vi "Initialize.vi"(8 "error in (no error)":errorcluster, 10 "Variable Names":string[](array[string]), 11 "Expression":string) -> (0 "error out":errorcluster, 3 "Expression":T1)   [LabVIEW 2022 SP3, in "Expressions.lvlib"]
uses:
  Expressions.lvlib
  Controls/Expression.ctl
  Controls/Token Type.ctl
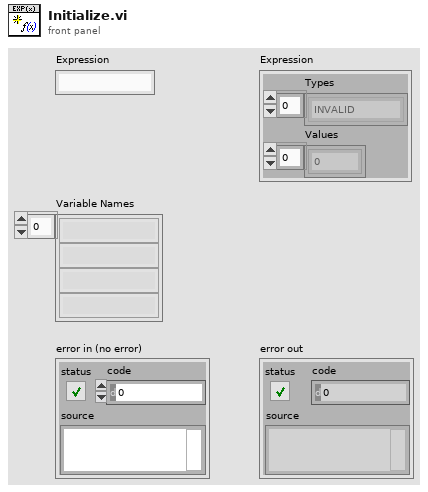
[diagram p1: front panel]
types:
  T1 = typedef "Expressions.lvlib/Expression.ctl" = cluster{"Types":T2[], "Values":dbl[]}
  T2 = typedef "Expressions.lvlib/Token Type.ctl" = enum8{"INVALID", "NOT", "AND", "OR", "EE", "NE", "LT", "GT", "LTE", "GTE", "PLUS", "MINUS", "MULTIPLY", "DIVIDE", "MODULUS", "LPAREN", "RPAREN", "LITERAL", "IDENTIFIER", "DEFINITION"}
  T3 = typedef "Expressions.lvlib/Token.ctl" = cluster{"Offset":i32, "Type":T2, "Value":string}
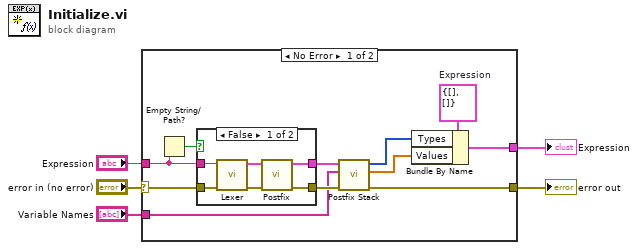
[diagram p0: block diagram]
diagram:
  n1 = case shown="No Error" "error in (no error)" {
    selector: "error in (no error)" -> [w16 w24]
    tunnel: "Expression" -> [w15 _]
    tunnel: "Variable Names" -> [w8 _]
    tunnel: [w10 w24] -> w2
    tunnel: [w12 _] -> w1
    frame No Error {
      w14 = T1 {"Types"=[], "Values"=[]}  # Expression
      n2 = Empty String/Path?(string/path=w15) -> (empty?=w13:bool)
      n3 = case shown="False" w13 {
        tunnel: [w22 w23] -> w11
        tunnel: w16 -> [w21 w23]
        tunnel: w15 -> [w20 _]
        tunnel: [w17 _] -> w9
        frame False {
          n4 = call "Lexer.vi"("error in (no error)"=w21, "Input"=w20) -> ("error out"=w19:errorcluster, "Tokens"=w18:T3[])  [unwired: 8 in]
          n5 = call "Postfix.vi"("error in (no error)"=w19, "Infix"=w18) -> ("error out"=w22:errorcluster, "Postfix"=w17:T3[])  [unwired: 8 in]
        }
        frame True {
        }
      }
      n6 = call "Postfix Stack.vi"("error in (no error)"=w11, "Variable Names"=w8, "Postfix"=w9) -> ("error out"=w10:errorcluster, "Values"=w6:dbl[], "Types"=w7:T2[])  [unwired: 6 in]
      n7 = Bundle By Name(cluster=w14, "Types"=w7, "Values"=w6) -> (w12:T1)
    }
    frame Error {
    }
  }
  "error out" <- w2
  "Expression" <- w1
